vi "Open Comm.vi"(8 "error in (no error)":errorcluster, 11 "AISAS Mech in":refnum<class "AISAS Mech.lvclass">) -> (0 "error out":errorcluster, 2 "Comm port ok?":bool, 3 "AISAS Mech out":refnum<class "AISAS Mech.lvclass">)   [LabVIEW 2014, in "AISAS Mech.lvclass"]
uses:
  AISAS Mech.lvclass
  AISAS Mech.lvclass/AISAS Mech.ctl
  motor/AISAS motor.lvclass/AISAS motor.ctl
  <vilib>/Instr/_visa.llb/VISA Configure Serial Port (Instr).vi
  motor/AISAS motor.lvclass
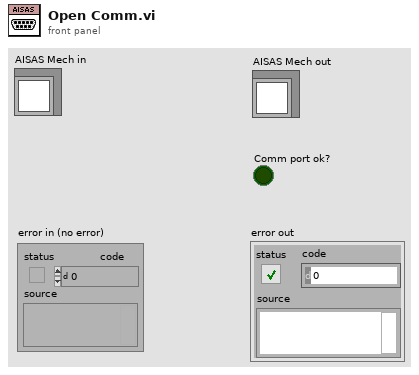
[diagram p1: front panel]
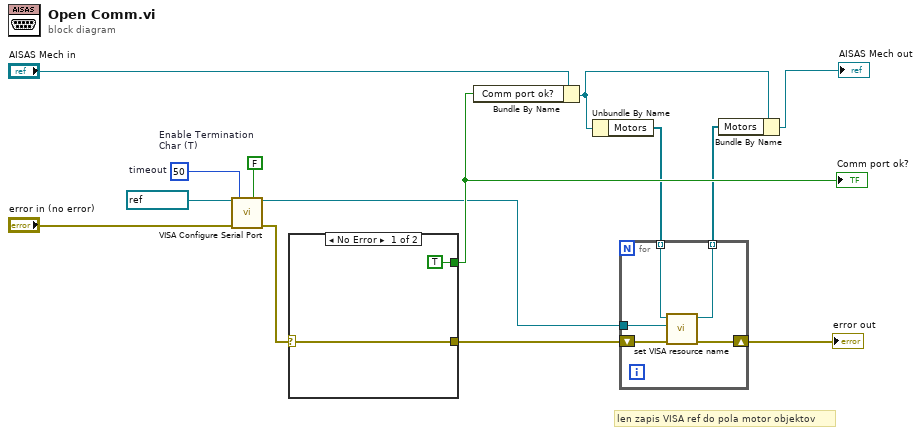
[diagram p0: block diagram]
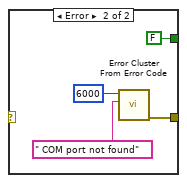
[diagram p2: hidden frame]
diagram:
  w11 = FALSE  # Enable Termination Char (T)
  w14 = u32 50  # timeout
  # "len zapis VISA ref do pola motor objektov"
  n1 = call-poly "VISA Configure Serial Port"("VISA resource name"=refnum<visa-resource-name> "COM7" ("VISA Refnum in"), "timeout (10sec)"=w14, "Enable Termination\nChar (T)"=w11, "error in (no error)"="error in (no error)") -> ("VISA resource name out"=w7:refnum<visa-resource-name>, "error out"=w12:errorcluster)  [unwired: 10 in]
  n2 = case shown="No Error" w12 {
    selector: w12 -> [w16 _]
    tunnel: [w16 w18] -> w3
    tunnel: [TRUE ("COM port ok?") FALSE ("COM port ok?")] -> w9
    frame No Error {
    }
    frame Error {
      n3 = call <vilib>:"Error Cluster From Error Code.vi"("error message (\"\")"=" COM port not found" ("error message (\"\")"), "error code (0)"=6000) -> ("error out"=w18:errorcluster)  [unwired: 7 in]
    }
  }
  "Comm port ok?" <- w9
  n4 = Bundle By Name(cluster="AISAS Mech in", "Comm port ok?"=w9) -> (w6:refnum<class "AISAS Mech.lvclass">)
  n5 = Unbundle By Name(w6) -> ("Motors"=w8:refnum<class "AISAS motor.lvclass">[])
  n6 = for {
    tunnel: w8 -> [w25] mode=indexing
    tunnel: w7 -> [w24]
    tunnel: [w23] -> w5 mode=indexing
    shift-right: [w22] -> w4
    shift-left: w3 -> [w21]
    n7 = call "set VISA resource name.vi"("error in (no error)"=w21, "VISA resource name"=w24, "AISAS motor in"=w25) -> ("error out"=w22:errorcluster, "AISAS motor out"=w23:refnum<class "AISAS motor.lvclass">)  [unwired: 7 in]
  }
  "error out" <- w4
  n8 = Bundle By Name(cluster=w6, "Motors"=w5) -> (→"AISAS Mech out":refnum<class "AISAS Mech.lvclass">)
